vi "SMC one step.vi"(8 "error in (no error)":errorcluster, 9 "Relative Step Size":dbl, 10 "Axis in":i32=1, 11 "VISA Handle in":refnum<visa-resource-name>) -> (0 "error out":errorcluster, 2 "Axis 2 (y axis)":dbl format="%.6f", 3 "Axis 1 x axis":dbl format="%.6f")   [LabVIEW 2012]
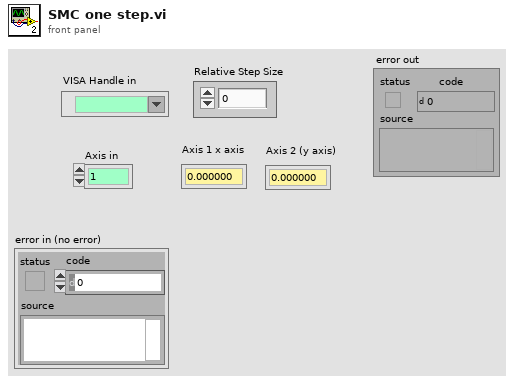
[diagram p1: front panel]
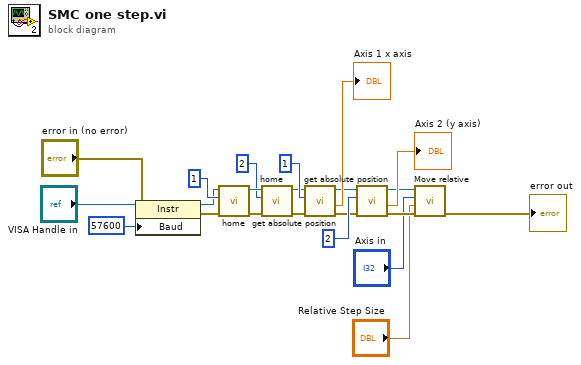
[diagram p0: block diagram]
diagram:
  n1 = property class="Instr"(reference="VISA Handle in", error in="error in (no error)", "Baud"=u32 57600 ("Serial Settings:Baud Rate")) -> (reference out=w17:refnum<visa-resource-name>, error out=w16:errorcluster)
  n2 = call "home.vi"("error in"=w16, "Axis in"=1, "VISA Handle in"=w17) -> ("error out"=w22:errorcluster, "VISA Handle out"=w21:refnum<visa-resource-name>)  [unwired: 3 in, 2 out]
  n3 = call "home.vi"("error in"=w22, "Axis in"=2, "VISA Handle in"=w21) -> ("error out"=w7:errorcluster, "VISA Handle out"=w8:refnum<visa-resource-name>)  [unwired: 3 in, 2 out]
  n4 = call "get absolute position.vi"("error in"=w7, "Axis in"=1, "VISA Handle in"=w8) -> ("error out"=w9:errorcluster, "Target position (units)"=→"Axis 1 x axis":dbl, "VISA Handle out"=w10:refnum<visa-resource-name>)  [unwired: 2 in, 2 out]
  n5 = call "get absolute position.vi"("error in"=w9, "Axis in"=2, "VISA Handle in"=w10) -> ("error out"=w5:errorcluster, "Target position (units)"=→"Axis 2 (y axis)":dbl, "VISA Handle out"=w6:refnum<visa-resource-name>)  [unwired: 2 in, 2 out]
  n6 = call "Move relative.vi"("error in"=w5, "Displacement (units)"="Relative Step Size", "Axis in"="Axis in", "VISA Handle in"=w6) -> ("error out"=→"error out":errorcluster)  [unwired: 2 in, 3 out]
